vi "GetAll__slk_tc.vi"(0 "tree control in":refnum<class "TreeControl.lvclass">, 5 "start tag":string, 9 "input tree items (do not wire)":string[](array[string]), 11 "error in (no error)":errorcluster) -> (4 "tree control out":refnum<class "TreeControl.lvclass">, 6 "current tag":string, 10 "output tree items":string[](array[string]), 15 "error out":errorcluster)   [LabVIEW 2020, in "TreeControl.lvclass"]
doc: "Retrieves all elements in tree at and below the starting tag. When Starting Tag and Input Tree Items are left unwired it will return all elements in the tree."
uses:
  Library/TreeControl.lvclass
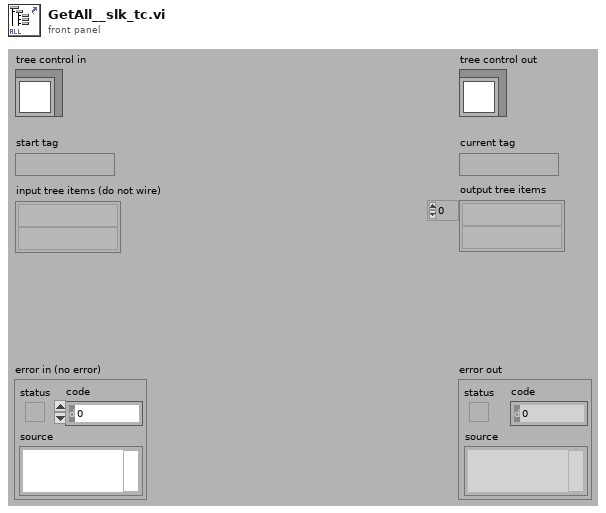
[diagram p1: front panel]
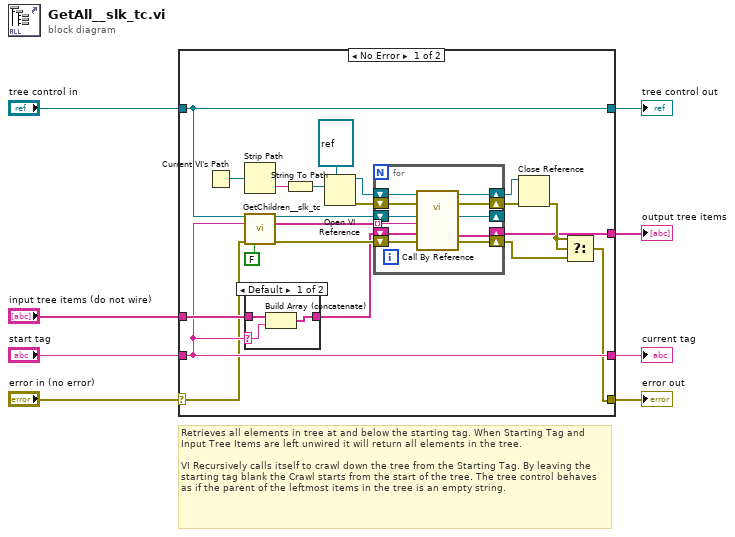
[diagram p0: block diagram]
diagram:
  # "Retrieves all elements in tree at and below the starting tag. When Starting Tag and Input Tree Items are left unwired it will return all elements in the tree. \n\nVI Recursively calls itself to crawl down the tree from the Starting Tag. By leaving the starting tag blank the Crawl starts from the start of the tree. The tree control behaves as if the parent of the leftmost items in the tree is an empty string."
  n1 = case shown="No Error" "error in (no error)" {
    selector: "error in (no error)" -> [w12 w46]
    tunnel: [w11 w46] -> w7
    tunnel: [w29 w45] -> w5
    tunnel: "tree control in" -> [w29 w45]
    tunnel: "start tag" -> [w13 _]
    tunnel: "input tree items (do not wire)" -> [w16 _]
    tunnel: [w14 _] -> w2
    tunnel: [w13 _] -> w1
    frame No Error {
      n2 = Current VI's Path() -> (path=w28:path)
      n3 = Strip Path(path=w28) -> (name=w27:string)  [unwired: 1 out]
      n4 = call "GetChildren__slk_tc.vi"("tree control in"=w29, "parent tag (\"\")"=w13, "error in (no error)"=w12, "use current (T)"=FALSE ("Use Current (T)")) -> ("tree control out"=w22:refnum<class "TreeControl.lvclass">, "children tags"=w24:string[], "error out"=w21:errorcluster)  [unwired: 9 out]
      n5 = case shown="Default" w13 {
        selector: w13 -> [w30 _]
        tunnel: w16 -> [w32 w33]
        tunnel: [w31 w33] -> w15
        frame Default {
          n6 = Build Array (concatenate)(w32, w30) -> (w31:string[])
        }
        frame "" {
        }
      }
      n7 = String To Path(string=w27) -> (path=w10:path)
      n8 = Open VI Reference(type specifier VI Refnum (for type only)=refnum<vi> refnum, vi path=w10) -> (vi reference=w25:refnum<vi>, error out=w23:errorcluster)  [unwired: 1 in, 3 out]
      n9 = for {
        tunnel: w24 -> [w39] mode=indexing
        shift-right: [w43] -> w19
        shift-left: w25 -> [w44]
        shift-right: [w41] -> w20
        shift-left: w23 -> [w42]
        shift-right: [w37] -> w14
        shift-left: w15 -> [w38]
        shift-right: [w34] -> _
        shift-left: w22 -> [w40]
        shift-right: [w35] -> w17
        shift-left: w21 -> [w36]
        n10 = call-by-ref "?"(reference=w44, error in=w42, "Tree Control in"=w40, "Start Tag"=w39, "Input Tree Items (DO NOT WIRE)"=w38, 11:"error in (no error)"=w36) -> (reference out=w43:refnum<vi>, error out=w41:errorcluster, "Tree Control out"=w34:refnum<class "TreeControl.lvclass">, "Output Tree Items"=w37:string[], 15:"error out"=w35:errorcluster)  [unwired: 8 in, 1 out]
      }
      n11 = Close Reference(reference=w19, error in (no error)=w20) -> (error out=w18:errorcluster)
      n12 = Select(t=w18, s=w18, f=w17) -> (s? t:f=w11:errorcluster)
    }
    frame Error {
    }
  }
  "error out" <- w7
  "tree control out" <- w5
  "output tree items" <- w2
  "current tag" <- w1
